vi "Create Data File.vi"(8 "错误输入":cluster{"状态":bool, "代码":i32, "源":string}) -> (0 "错误输出":cluster{"状态":bool, "代码":i32, "源":string}, 3 "文件引用句柄":refnum<file>)   [LabVIEW 2012]
doc: "本VI通过执行一系列任务，为记录数据创建一个文件：\n\n1) 检查应用程序目录下是否存在名称为Logged Data的文件夹\n2) 如不存在，则创建该文件夹\n3) 按“采集数据 <日期> <时间>.txt”格式，生成一个文件名称\n4) 替换或创建文件"
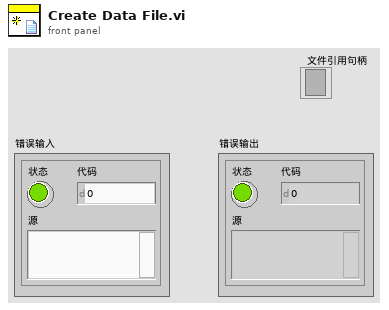
[diagram p1: front panel]
types:
  T1 = enum16{"open", "replace", "create", "open or create", "replace or create", "replace or create with confirmation"}
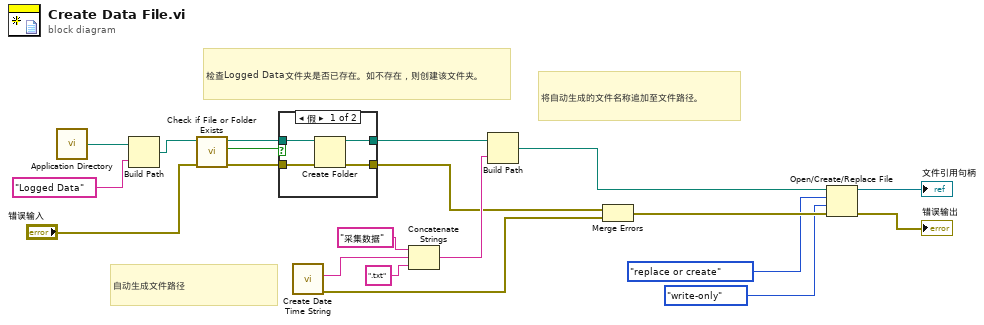
[diagram p0: block diagram]
diagram:
  # "将自动生成的文件名称追加至文件路径。"
  # "检查Logged Data文件夹是否已存在。如不存在，则创建该文件夹。"
  # "自动生成文件路径"
  n1 = call <vilib>:"Application Directory.vi"() -> ("Application Directory"=w1:path)
  n2 = Build Path ("创建路径")(base path=w1, name or relative path="Logged Data" ("对话框窗口（创建文件夹）")) -> (appended path=w5:path)
  n3 = call <vilib>:"Check if File or Folder Exists.vi"("error in (no error)"="错误输入", "path"=w5) -> ("error out"=w4:errorcluster, "file or folder exists?"=w2:bool, "dup path"=w3:path)  [unwired: 7 in]
  n4 = case shown="假" w2 {
    tunnel: [w24 w26] -> w13
    tunnel: [w23 w25] -> w8
    tunnel: w4 -> [w22 w25]
    tunnel: w3 -> [w21 w26]
    frame False {
      n5 = Create Folder ("创建文件夹")(path (use dialog)=w21, error in=w22) -> (created path=w24:path, error out=w23:errorcluster)  [unwired: 1 in, 1 out]
    }
    frame True {
    }
  }
  n6 = call "Create Date Time String.vi"() -> ("错误输出"=w7:cluster{"状态":bool, "代码":i32, "源":string}, "日期/时间字符串"=w11:string)  [unwired: 10 in]
  n7 = Concatenate Strings ("连接字符串")("采集数据" ("字符串"), w11, ".txt" ("字符串")) -> (w9:string)
  n8 = Build Path ("创建路径")(base path=w13, name or relative path=w9) -> (appended path=w20:path)
  n9 = Merge Errors ("合并错误")(w8, w7) -> (w19:errorcluster)
  n10 = Open/Create/Replace File ("打开/创建/替换文件")(file path (use dialog)=w20, error in=w19, operation (0:open)=T1."replace or create" ("操作(0:open)"), access (0:read/write)=enum16{"read/write", "read-only", "write-only"}."write-only" ("权限(0:read/write)")) -> (refnum out=→"文件引用句柄":refnum<file>, error out=→"错误输出":errorcluster)  [unwired: 2 in, 1 out]
